vi "Database Query Search With Return Value.vi"(8 "error in (no error)":errorcluster, 10 "SQL query":string, 11 "object in":refnum<class "DatabaseAPI.lvclass">) -> (0 "error out":errorcluster, 1 "Not Empty":bool, 2 "recordset data":variant[][](array[variant]), 3 "object out":refnum<class "DatabaseAPI.lvclass">)   [LabVIEW 2015, in "DatabaseAPI.lvclass"]
uses:
  DatabaseAPI.lvclass
  <vilib>/addons/database/Auxilliary.llb/DB Tools Cursor Type.ctl
  DatabaseAPI.lvclass/DatabaseAPI.ctl
  <vilib>/addons/database/Connection.llb/DB Tools Open Connec (String).vi
  <vilib>/addons/database/Connection.llb/Conn Execute.vi
  <vilib>/addons/database/Recordset.llb/Rec Get Recordset Properties (R).vi
  <vilib>/addons/database/Recordset.llb/Rec Fetch Recordset Data (R).vi
  <vilib>/addons/database/Recordset.llb/Rec Destroy - Connection.vi
  <vilib>/addons/database/NI_Database_API.lvlib
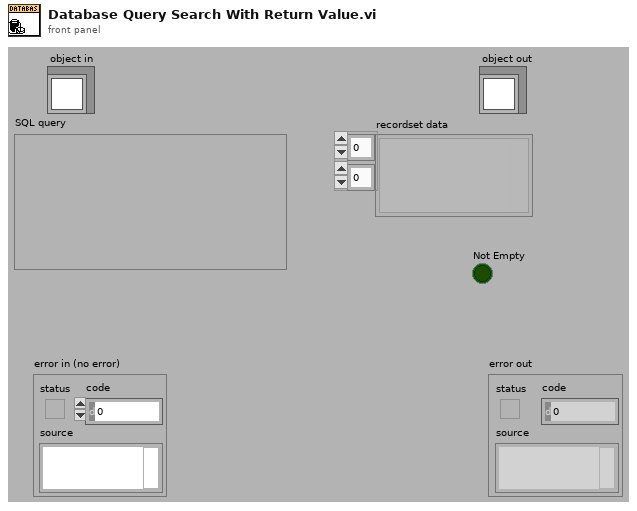
[diagram p1: front panel]
types:
  T1 = typedef "NI_Database_API.lvlib/DB Tools Cursor Type.ctl" = enum16{"forward-only", "keyset", "dynamic", "static"}
  T2 = typedef "NI_Database_API.lvlib/Conn ObjectReference.ctl" = refnum<k1>
  T3 = typedef "NI_Database_API.lvlib/Rec ObjectReference.ctl" = refnum<k1>
  T4 = typedef "NI_Database_API.lvlib/Rec Properties.ctl" = cluster{"column count":i32, "record index":i32, "record count":i32, "bof?":bool, "eof?":bool, "cursor type":T1, "cache size":i32, "state":enum16{"closed", "open"}}
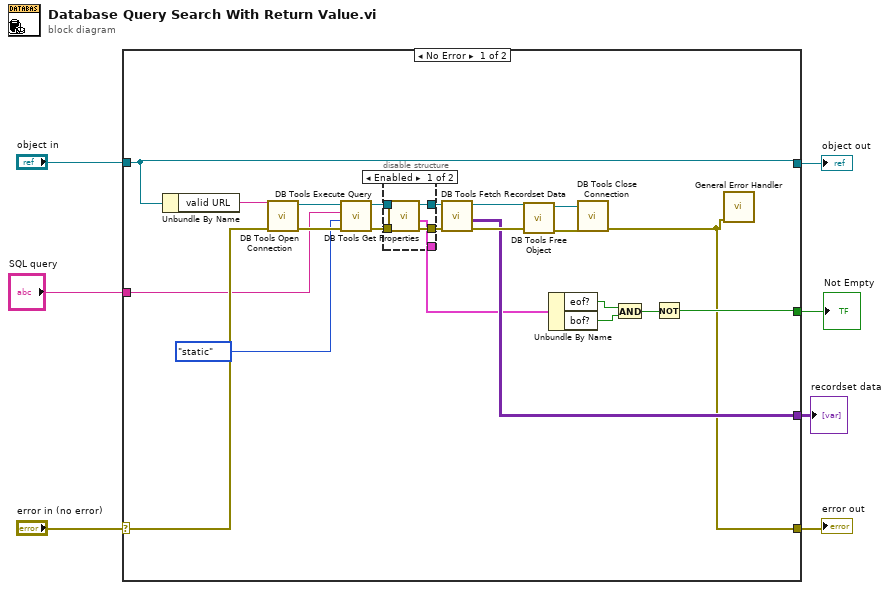
[diagram p0: block diagram]
diagram:
  n1 = case shown="No Error" "error in (no error)" {
    selector: "error in (no error)" -> [w27 w38]
    tunnel: [w8 w38] -> w6
    tunnel: [w29 w37] -> w4
    tunnel: "object in" -> [w29 w37]
    tunnel: "SQL query" -> [w23 _]
    tunnel: [w18 _] -> w2
    tunnel: [w9 _] -> w1
    frame No Error {
      n2 = Unbundle By Name(w29) -> ("valid URL"=w28:string)
      n3 = call-poly <vilib>:"DB Tools Open Connection.vi"("error in (no error)"=w27, "connection information"=w28) -> ("error out"=w25:errorcluster, "connection reference"=w26:T2)  [unwired: 6 in]
      n4 = call-poly <vilib>:"DB Tools Execute Query.vi"("error in (no error)"=w25, "cursor type"=DB_Tools_Cursor_Type."static", "SQL query"=w23, "connection reference"=w26) -> ("error out"=w16:errorcluster, "recordset reference"=w17:T3)  [unwired: 4 in]
      n5 = disable-structure shown="Enabled" {
        disable-tunnel: w17 -> [w34 w36]
        disable-tunnel: w16 -> [w33 w35]
        disable-tunnel: [w32 w36] -> w15
        disable-tunnel: [w31 w35] -> w14
        disable-tunnel: [w30 _] -> w13
        frame Enabled {
          n6 = call-poly <vilib>:"DB Tools Get Properties.vi"("error in (no error)"=w33, "recordset reference"=w34) -> ("error out"=w31:errorcluster, "recordset properties"=w30:T4, "recordset reference out"=w32:T3)  [unwired: 3 in]
        }
        frame Disabled {
        }
      }
      n7 = call-poly <vilib>:"DB Tools Fetch Recordset Data.vi"("error in (no error)"=w14, "recordset reference"=w15) -> ("error out"=w19:errorcluster, "recordset data"=w18:variant[][], "recordset reference out"=w20:T3)  [unwired: 3 in]
      n8 = call-poly <vilib>:"DB Tools Free Object.vi"("error in (no error)"=w19, "recordset reference"=w20) -> ("error out"=w22:errorcluster, "connection reference"=w21:T2)  [unwired: 8 in]
      n9 = Unbundle By Name(w13) -> ("eof?"=w12:bool, "bof?"=w11:bool)
      n10 = call <vilib>:"DB Tools Close Connection.vi"("error in (no error)"=w22, "connection reference"=w21) -> ("error out"=w8:errorcluster)  [unwired: 5 in]
      n11 = And(x=w12, y=w11) -> (x .and. y?=w10:bool)
      n12 = Not(x=w10) -> (.not. x?=w9:bool)
      n13 = call <vilib>:"General Error Handler.vi"("error in (no error)"=w8) -> ()  [unwired: 10 in, 5 out]
    }
    frame Error {
    }
  }
  "error out" <- w6
  "object out" <- w4
  "recordset data" <- w2
  "Not Empty" <- w1
